vi "Send Data Message.vi"(8 "error in (no error)":errorcluster, 10 "data string":string, 11 "Message Enqueuer in":refnum<class "Message Enqueuer.lvclass">) -> (0 "error out":errorcluster)   [LabVIEW 2016, in "Assert API Components.lvlib" / "Assert Service.lvlib" / "Assert Service.lvclass"]
uses:
  Assert Service.lvclass
  <vilib>/ActorFramework/Message Enqueuer/Message Enqueuer.lvclass
  Main Display/Main Display Messages/New Assert Message Msg/New Assert Message Msg.lvclass/New Assert Message Msg.ctl
  <vilib>/ActorFramework/Message Enqueuer/Message Enqueuer.lvclass/Message Enqueuer.ctl
  <vilib>/ActorFramework/Message Enqueuer/Enqueue.vi
  Main Display/Main Display Messages/New Assert Message Msg/New Assert Message Msg.lvclass
  C:/Program Files (x86)/National Instruments/LabVIEW 2016/vi.lib/ActorFramework/Message/Message.lvclass
  <vilib>/ActorFramework/Message Priority Queue/Priority Enqueue.vi
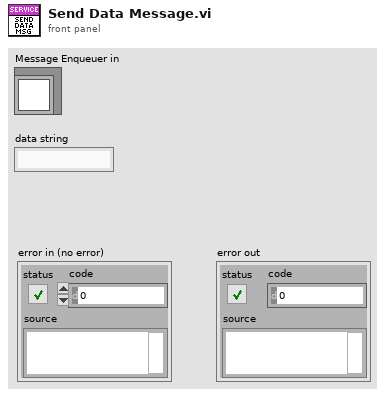
[diagram p1: front panel]
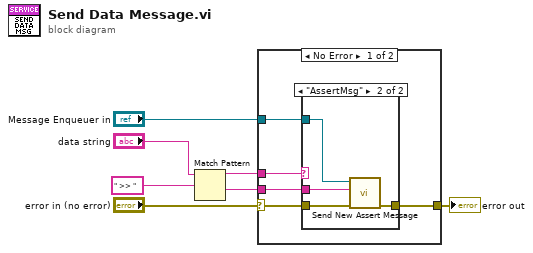
[diagram p0: block diagram]
diagram:
  n1 = Match Pattern(string="data string", regular expression=" >> " ("Msg Name")) -> (before substring=w1:string, after substring=w2:string)  [unwired: 1 in, 2 out]
  n2 = case shown="No Error" "error in (no error)" {
    selector: "error in (no error)" -> [w10 w18]
    tunnel: [w12 w18] -> w7
    tunnel: "Message Enqueuer in" -> [w11 _]
    tunnel: w2 -> [w9 _]
    tunnel: w1 -> [w8 _]
    frame No Error {
      n3 = case shown="\"AssertMsg\"" w8 {
        tunnel: [w13 w17] -> w12
        tunnel: w10 -> [w13 w16]
        tunnel: w9 -> [_ w15]
        tunnel: w11 -> [_ w14]
        frame Default {
        }
        frame "AssertMsg" {
          n4 = call "Send New Assert Message.vi"("error in (no error)"=w16, "Assert Message"=w15, "Message Enqueuer"=w14) -> ("error out"=w17:errorcluster)  [unwired: 7 in, 1 out]
        }
      }
    }
    frame Error {
    }
  }
  "error out" <- w7
